vi "Adjust Record Baselines.vi"(1 "Extension Baseline (nm)":dbl, 2 "Force Baseline (pN)":dbl, 3 "Record":T1) -> (0 "Adjusted Record":T1)   [LabVIEW 2013]
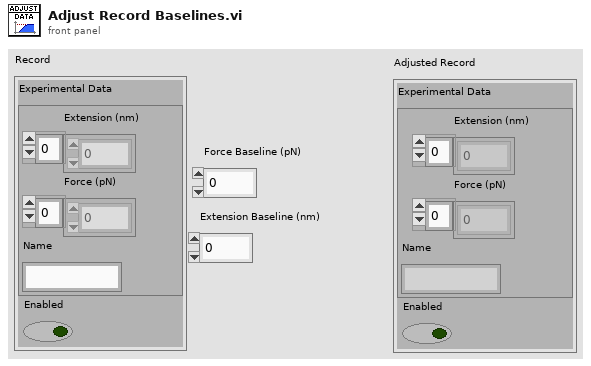
[diagram p1: front panel]
types:
  T1 = cluster{"Experimental Data":cluster{"Extension (nm)":dbl[], "Force (pN)":dbl[], "Name":string}, "Enabled":bool}
  T2 = cluster{"Extension (nm)":dbl[], "Force (pN)":dbl[], "Name":string}
  T3 = cluster{cluster{dbl[], dbl[], "Name":string}, "Enabled":bool}
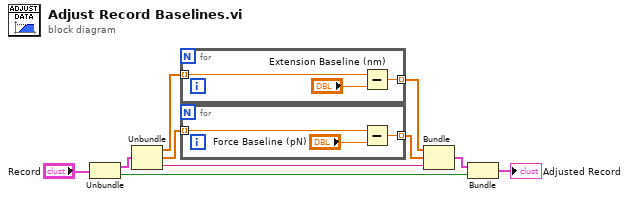
[diagram p0: block diagram]
diagram:
  n1 = Unbundle("Record") -> ("Experimental Data"=w3:T2, "Enabled"=w10:bool)
  n2 = Unbundle(w3) -> ("Extension (nm)"=w4:dbl[], "Force (pN)"=w5:dbl[], "Name"=w8:string)
  n3 = for {
    tunnel: w4 -> [w13] mode=indexing
    tunnel: [w12] -> w6 mode=indexing
    n4 = Subtract(x=w13, y="Extension Baseline (nm)") -> (x-y=w12:dbl)
  }
  n5 = for {
    tunnel: w5 -> [w16] mode=indexing
    tunnel: [w15] -> w7 mode=indexing
    n6 = Subtract(x=w16, y="Force Baseline (pN)") -> (x-y=w15:dbl)
  }
  n7 = Bundle(w6, w7, "Name"=w8) -> (w9:cluster{dbl[], dbl[], "Name":string})  [unwired: 1 in]
  n8 = Bundle(w9, "Enabled"=w10) -> (→"Adjusted Record":T3)  [unwired: 1 in]
